vi "Connector1 Digital Input.vi"() -> (0 "Packet":u64)   [LabVIEW 2010]
uses:
  <vilib>/eio/EIONode/EIONode.xnode
  <vilib>/rvi/eio/nirviEIOImplementation/nirviEIOImplementation.xnode
  <vilib>/rvi/eio/common/nirviEmuClasses.ctl
  <vilib>/rvi/eio/common/nirviEmuTemplateMethod_noerrors.vi
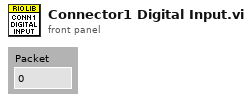
[diagram p1: front panel]
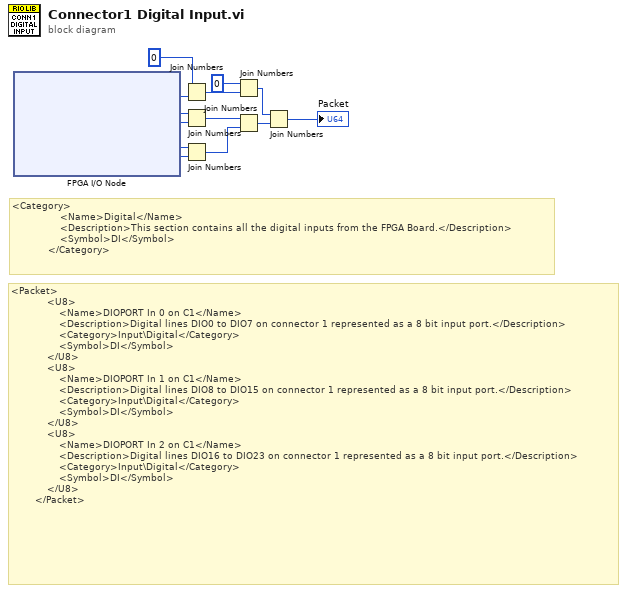
[diagram p0: block diagram]
diagram:
  # "<Packet>\n            <U8>\n                <Name>DIOPORT In 0 on C1</Name>\n                <Description>Digital lines DIO0 to DIO7 on connector 1 represented as a 8 bit input port.</Description>\n                <Category>Input\\Digital</Category>\n                <Symbol>DI</Symbol>\n            </U8>\n            <U8>\n                <Name>DIOPORT In 1 on C1</Name>\n                <Description>Digital lines DIO8 to DIO15 on connector 1 represented as a 8 bit input port.</Description>\n                <Category>Input\\Digital</Category>\n                <Symbol>DI</Symbol>\n            </U8>\n            <U8>\n                <Name>DIOPORT In 2 on C1</Name>\n                <Description>Digital lines DIO16 to DIO23 on connector 1 represented as a 8 bit input port.</Description>\n                <Category>Input\\Digital</Category>\n                <Symbol>DI</Symbol>\n            </U8>\n        </Packet>"
  # "<Category>\n                <Name>Digital</Name>\n                <Description>This section contains all the digital inputs from the FPGA Board.</Description>\n                <Symbol>DI</Symbol>\n            </Category>"
  n1 = xnode "FPGA I/O Node"() -> ("Connector1/DIOPORT4"=w1:u8, "Connector1/DIOPORT3"=w2:u8, "Connector1/DIOPORT2"=w3:u8, "Connector1/DIOPORT1"=w4:u8, "Connector1/DIOPORT0"=w5:u8)  [unwired: 5 in, 5 out]
  n2 = Join Numbers(hi=u8 0, lo=w1) -> ((hi.lo)=w6:u16)
  n3 = Join Numbers(hi=w2, lo=w3) -> ((hi.lo)=w7:u16)
  n4 = Join Numbers(hi=w4, lo=w5) -> ((hi.lo)=w8:u16)
  n5 = Join Numbers(hi=u16 0, lo=w6) -> ((hi.lo)=w9:u32)
  n6 = Join Numbers(hi=w7, lo=w8) -> ((hi.lo)=w10:u32)
  n7 = Join Numbers(hi=w9, lo=w10) -> ((hi.lo)=→"Packet":u64)
